vi "histogram.vi"(1 "Array":i32[](array[numeric])) -> (0 "Histogram":picture)   [LabVIEW 2017]
uses:
  <vilib>/picture/cartesn2.llb/Waveform Plot Type.ctl
panel:
  in  "Numeric 2":dbl=1.0 format="%#_13g"
  in  "Numeric":dbl=0.5 format="%#_13g"
  in  "cartesian grid cosmetics":T1={"line color"=39168, "text color"=65280, "tick length(3)"=3, "crossing axes"=FALSE, "visible grid?"=TRUE}
  in  "waveform plot cosmetics":T3={"plot color"=5064, "plot type"=enum."bar plot", "baseline"=0.0}
  in  "cartesian axis attributes":T4={"x minimum"=0.0, "x maximum"=0.0, "x log?"=FALSE, "x precision"=1, "x format"=enum."Decimal", "y minimum"=0.0, "y maximum"=0.0, "y log?"=FALSE, "y precision"=1, "y format"=enum."Decimal"}
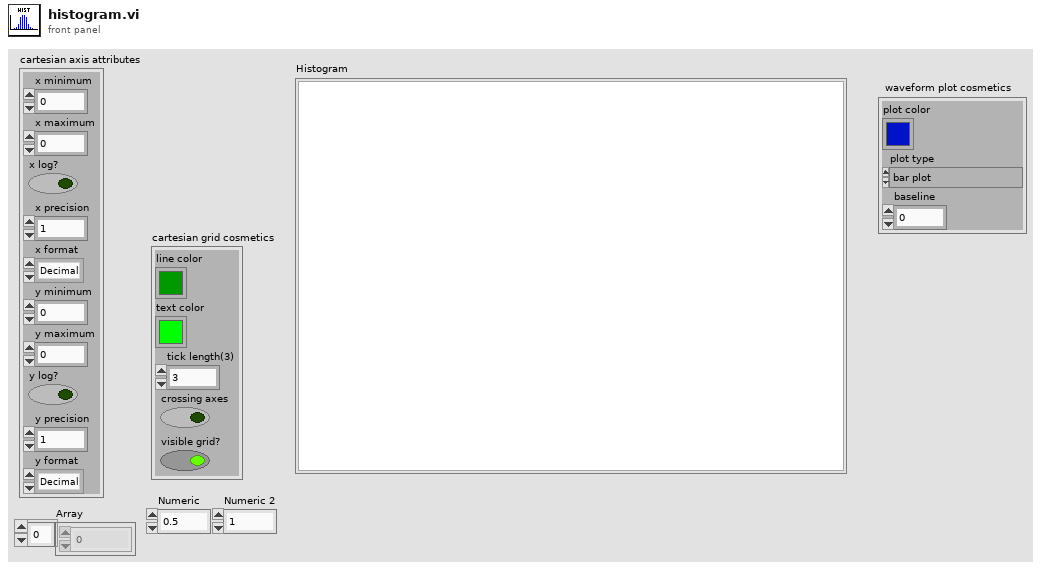
[diagram p1: front panel]
types:
  T1 = cluster{"line color":u32, "text color":u32, "tick length(3)":i16, "crossing axes":bool, "visible grid?":bool}
  T2 = typedef "Waveform Plot Type.ctl" = enum16{"points", "squares", "circles", "connected points", "connected squares", "connected circles", "fill to baseline", "comb plot", "bar plot"}
  T3 = cluster{"plot color":u32, "plot type":T2, "baseline":dbl}
  T4 = cluster{"x minimum":dbl, "x maximum":dbl, "x log?":bool, "x precision":u8, "x format":enum8{"Decimal", "Scientific", "Engineering", "Binary", "Octal", "Hex"}, "y minimum":dbl, "y maximum":dbl, "y log?":bool, "y precision":u8, "y format":enum8{"Decimal", "Scientific", "Engineering", "Binary", "Octal", "Hex"}}
  T5 = typedef "LVBoundsTypeDef.ctl" = cluster{"Width":u32, "Height":u32}
  T6 = cluster{"Numeric":dbl, "Numeric 2":dbl, "Array":i32[]}
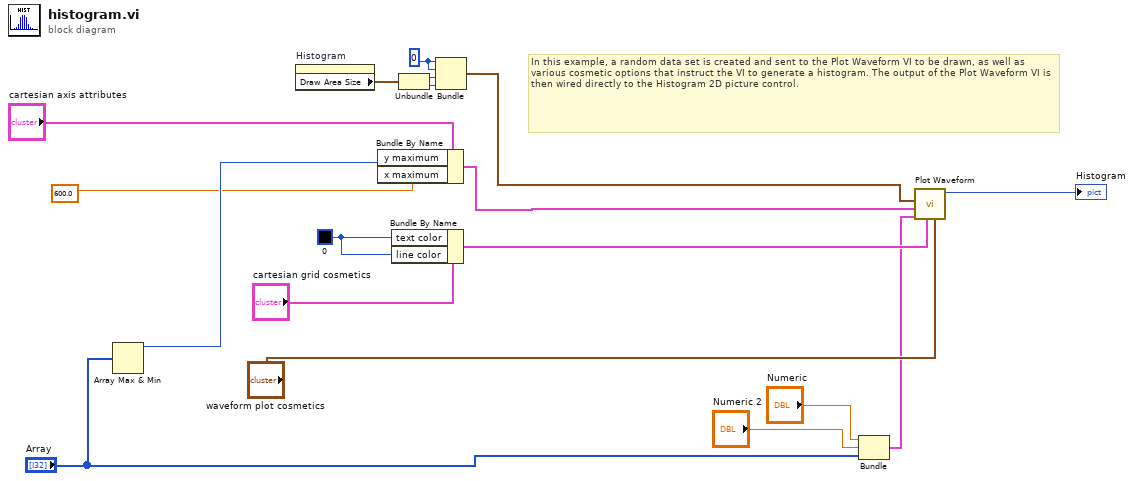
[diagram p0: block diagram]
diagram:
  w9 = u32 0
  w15 = 0
  # "In this example, a random data set is created and sent to the Plot Waveform VI to be drawn, as well as various cosmetic options that instruct the VI to generate a histogram. The output of the Plot Waveform VI is then wired directly to the Histogram 2D picture control."
  n1 = Array Max & Min(array="Array") -> (max value=w2:i32)  [unwired: 3 out]
  n2 = property on="Histogram" class="Pict"() -> ("Draw Area Size"=w18:T5)  [unwired: 2 in, 2 out]
  n3 = Bundle By Name(cluster="cartesian axis attributes", "y maximum"=w2, "x maximum"=600.0) -> (w8:T4)
  n4 = Bundle By Name(cluster="cartesian grid cosmetics", "text color"=w9, "line color"=w9) -> (w10:T1)
  n5 = Unbundle(w18) -> ("Width"=w16:u32, "Height"=w17:u32)
  n6 = Bundle(w15, w15, "Width"=w16, "Height"=w17) -> (w14:cluster{i32, i32, "Width":u32, "Height":u32})  [unwired: 1 in]
  n7 = Bundle("Numeric"="Numeric", "Numeric 2"="Numeric 2", "Array"="Array") -> (w7:T6)  [unwired: 1 in]
  n8 = call <vilib>:"Plot Waveform.vi"("waveform plot cosmetics"="waveform plot cosmetics", "cartesian grid cosmetics"=w10, "waveform data"=w7, "cartesian axis attributes"=w8, "bounding rect"=w14) -> ("new picture"=→"Histogram":picture)  [unwired: 6 in]
